vi "FindClosestAfter.vi"(2 "Setpoint":dbl, 3 "Sorted Array":dbl[](array[numeric])) -> (0 "Valid?":bool, 1 "Index next to setpoint":i32)   [LabVIEW 2016]
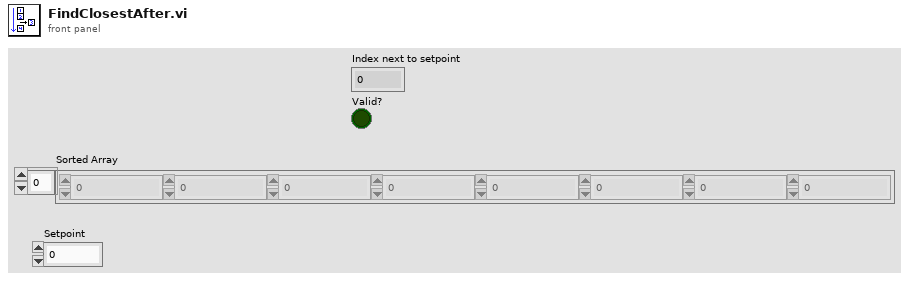
[diagram p1: front panel]
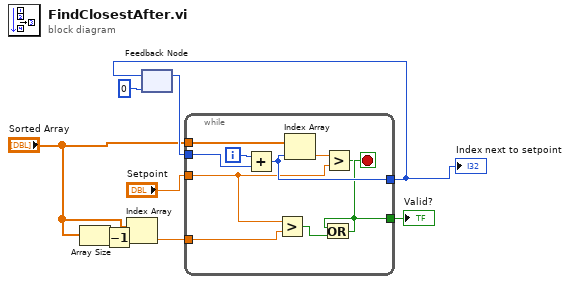
[diagram p0: block diagram]
diagram:
  n1 = Array Size(array="Sorted Array") -> (size(s)=w5:i32)
  n2 = Decrement(x=w5) -> (x-1=w1:i32)
  n3 = Index Array(array="Sorted Array", index=w1) -> (element=w3:dbl)
  n4 = feedback #1(0) -> (w8:i32)
  n5 = while {
    tunnel: "Sorted Array" -> [w19]
    tunnel: "Setpoint" -> [w14]
    tunnel: [w15] -> w6
    tunnel: w8 -> [w17]
    tunnel: w3 -> [w13]
    tunnel: [w10] -> w2
    i -> [w16]
    stop <- w11 stop-if-true
    n6 = Add(x=w16, y=w17) -> (x+y=w15:i32)
    n7 = Greater?(x=w14, y=w13) -> (0:w12:bool)
    n8 = Index Array(array=w19, index=w15) -> (element=w18:dbl)
    n9 = Greater?(x=w18, y=w14) -> (0:w10:bool)
    n10 = Or(x=w10, y=w12) -> (x .or. y?=w11:bool)
  }
  "Index next to setpoint" <- w6
  "Valid?" <- w2
  n11 = feedback-in #1(w6) -> ()
